vi "Report Plotter Test Interface.vi"() -> ()   [LabVIEW 2012, in "Report.lvlib"]
uses:
  Report.lvlib
panel:
  in  "Stop":bool
  in  "Plot":bool
  out "Report":path
  out "error out":errorcluster
  in  "error in":errorcluster
  out "Resistance":dynamicdata(graph)
  out "Pressure":dynamicdata(graph)
  out "Depth":dynamicdata(graph)
  out "Holding Potential":dynamicdata(graph)
  out "Current":dynamicdata(graph)
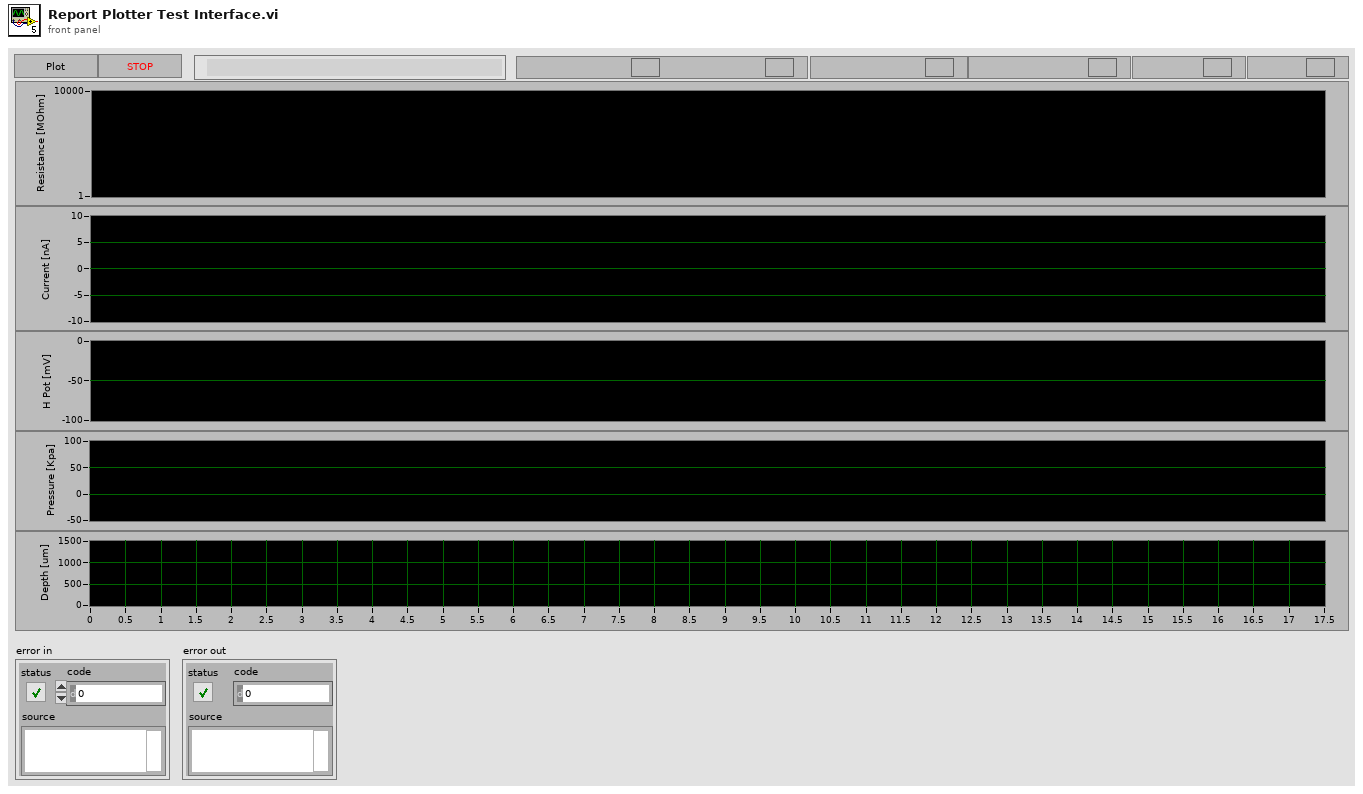
[diagram p1: front panel]
types:
  T1 = cluster{"Resistance":refnum<vi>, "Current":refnum<vi>, "Pressure":refnum<vi>, "Holding Potential":refnum<vi>, "Depth":refnum<vi>}
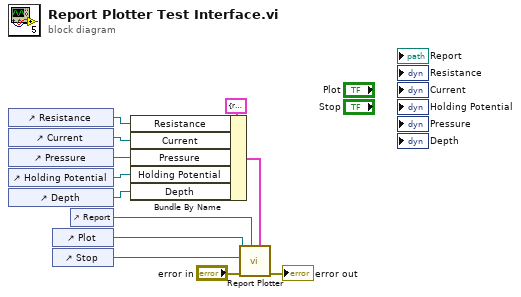
[diagram p0: block diagram]
diagram:
  n1 = control-ref of="Resistance"() -> (w9:refnum<vi>)
  n2 = control-ref of="Current"() -> (w8:refnum<vi>)
  n3 = control-ref of="Pressure"() -> (w7:refnum<vi>)
  n4 = control-ref of="Holding Potential"() -> (w6:refnum<vi>)
  n5 = control-ref of="Depth"() -> (w5:refnum<vi>)
  n6 = control-ref of="Plot"() -> (w1:refnum<vi>)
  n7 = control-ref of="Stop"() -> (w2:refnum<vi>)
  n8 = control-ref of="Report"() -> (w3:refnum<vi>)
  n9 = Bundle By Name(cluster=T1 {"Resistance"=refnum, "Current"=refnum, "Pressure"=refnum, "Holding Potential"=refnum, "Depth"=refnum} ("Indicators"), "Resistance"=w9, "Current"=w8, "Pressure"=w7, "Holding Potential"=w6, "Depth"=w5) -> (w4:T1)
  n10 = call "Report Plotter.vi"("Indicators"=w4, "Path"=w3, "error in"="error in", "Stop"=w2, "Plot"=w1) -> ("error out"=→"error out":errorcluster)  [unwired: 6 in]
